vi "Initialize Ref DAQ values.vi"(8 "error in (no error)":errorcluster, 10 "DAQ Input Parameters(FlexRIO)":T2 {"diff_threshZ" format="%#_11g"; "proportioanl_scale Z" format="%#_15g"; "var_x" format="%#_14g"; "var_y" format="%#_14g"; "scale" format="%#_15g"; "diff_thresh" format="%#_11g"; "proportioanl_scale" format="%#_15g"}, 11 "Refnum in":T1) -> (0 "error out":errorcluster, 3 "Refnum out":T1)   [LabVIEW 2020]
uses:
  RIG-SPECIFIC FILES/FPGA Refs/FPGA Ref.ctl
  <vilib>/rvi/interface/nirviReadWriteControl/nirviReadWriteControl.xnode
  <vilib>/rvi/interface/nirviMethod/nirviMethod.xnode
  NiFpgaLv.dll
  <vilib>/Utility/error.llb/Error Cluster From Error Code.vi
  <vilib>/rvi/interface/Simulation/niFpgaSimulationCallBeginRW.vi
  <vilib>/rvi/errors/niLvFpgaAdjustHostInterfaceError.vi
  <vilib>/FPGAPlugInAG/Dynamic/niLvFpga_StartFifo_Dynamic.vi
  <vilib>/rvi/errors/niLvFpgaMergeErrorWithErrorCode.vi
  FPGA DAQ/FPGA Typedefs/scan_typr.ctl
  Movement Correction/Typedefs/Control algorithm.ctl
  Typedefs/Controls/DAQ Input Parameters(FlexRIO).ctl
panel:
  out "scale":fxp<+,16,2>=1.0 format="%#_15g"
  out "New line trigger enabled":bool
  out "Ref count reset enabled":bool
  out "scan_int":fxp<+,16,2>
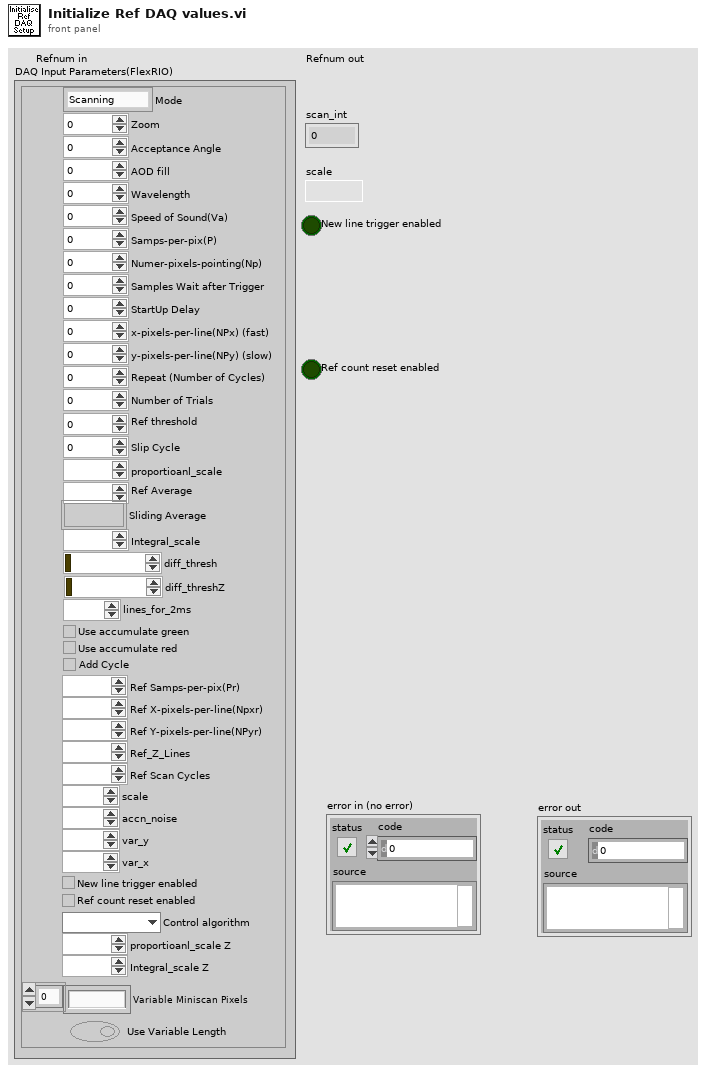
[diagram p1: front panel]
types:
  T1 = typedef "FPGA Ref.ctl" = refnum<k20>
  T2 = typedef "DAQ Input Parameters(FlexRIO).ctl" = cluster{"Mode":T3, "Zoom":i8, "Acceptance Angle":i8, "AOD fill":u16, "Wavelength":i16, "Speed of Sound(Va)":i8, "Samps-per-pix(P)":i16, "Numer-pixels-pointing(Np)":u32, "Samples Wait after Trigger":u16, "StartUp Delay":i32, "x-pixels-per-line(NPx) (fast)":u16, "y-pixels-per-line(NPy) (slow)":u16, "Repeat (Number of Cycles)":u32, "Number of Trials":u16, "Ref threshold":u16, "Slip Cycle":u32, "proportioanl_scale":fxp<+,16,2>, "Ref Average":u16, "Sliding Average":bool, "Integral_scale":fxp<+/-,16,12>, "diff_thresh":fxp<+/-,16,8>, "diff_threshZ":fxp<+/-,16,8>, "lines_for_2ms":i16, "Use accumulate green":bool, "Use accumulate red":bool, "Add Cycle":bool, "Ref Samps-per-pix(Pr)":i16, "Ref X-pixels-per-line(Npxr)":i16, "Ref Y-pixels-per-line(NPyr)":i16, "Ref_Z_Lines":i16, "Ref Scan Cycles":i32, "scale":fxp<+,16,2>, "accn_noise":fxp<+,16,16>, "var_y":fxp<+,16,4>, "var_x":fxp<+,16,4>, "New line trigger enabled":bool, "Ref count reset enabled":bool, "Control algorithm":T4, "proportioanl_scale Z":fxp<+,16,2>, "Integral_scale Z":fxp<+/-,16,12>, "Variable Miniscan Pixels":u16[], "Use Variable Length":bool}
  T3 = typedef "scan_typr.ctl" = enum16{"Scanning", "Pointing", "Pointing & MC", "Scanning & MC"}
  T4 = typedef "Control algorithm.ctl" = enum16{"PID", "Kalman"}
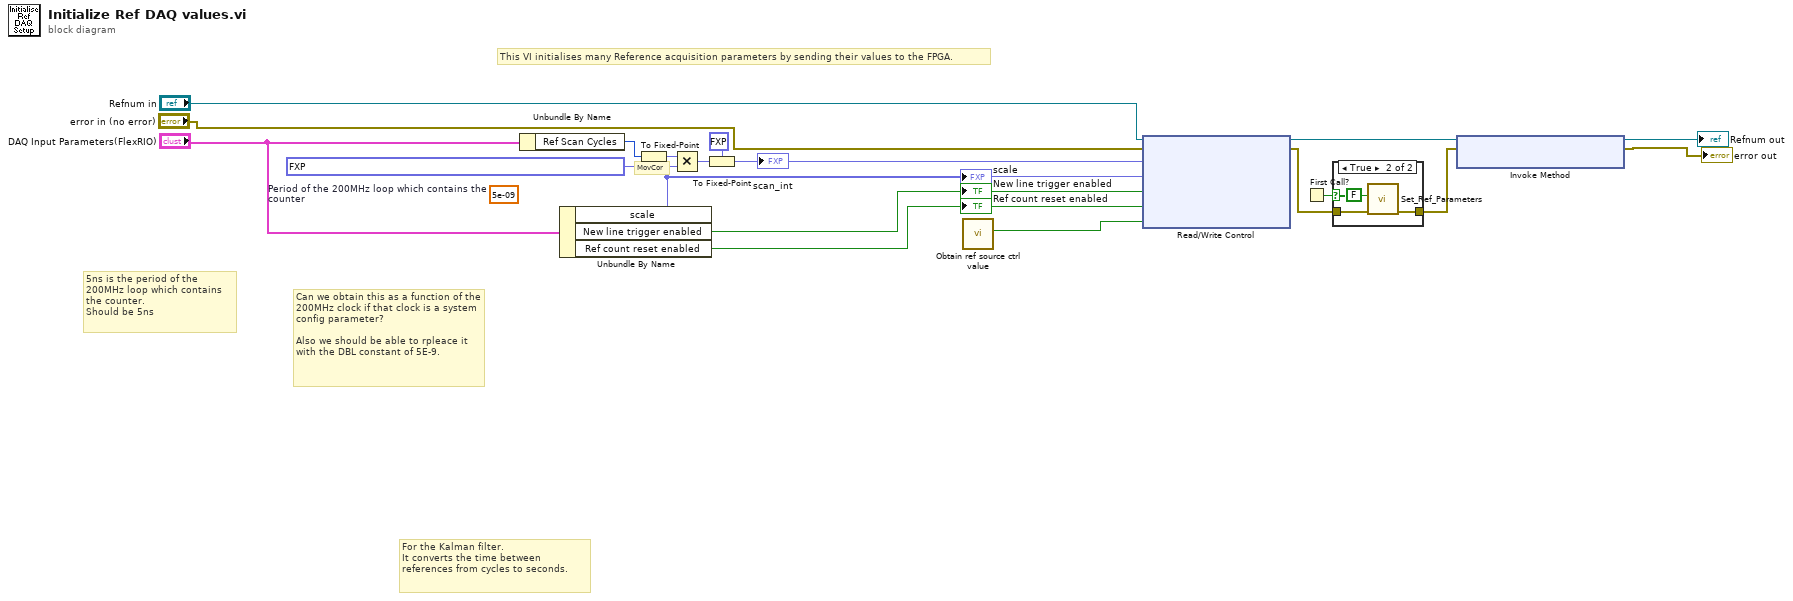
[diagram p0: block diagram]
diagram:
  (unwired) 5e-09  # Period of the 200MHz loop which contains the counter
  # "Can we obtain this as a function of the 200MHz clock if that clock is a system config parameter?\n\nAlso we should be able to rpleace it with the DBL constant of 5E-9."
  # "This VI initialises many Reference acquisition parameters by sending their values to the FPGA."
  # "MovCor"
  # "5ns is the period of the 200MHz loop which contains the counter.\nShould be 5ns"
  # "For the Kalman filter.\nIt converts the time between references from cycles to seconds."
  n1 = Unbundle By Name("DAQ Input Parameters(FlexRIO)") -> ("Ref Scan Cycles"=w12:i32)
  n2 = Unbundle By Name("DAQ Input Parameters(FlexRIO)") -> ("scale"=w14:fxp<+,16,2>, "New line trigger enabled"=w15:bool, "Ref count reset enabled"=w16:bool)
  "Ref count reset enabled" <- w16
  "New line trigger enabled" <- w15
  "scale" <- w14
  n3 = To Fixed-Point(number=w12) -> (fixed-point=w8:fxp<+/-,32,32>)  [unwired: 1 in]
  n4 = Multiply(x=w8, y=fxp<+,64,2> 4.999999999970306e-09 ("fixed-point type")) -> (x*y=w9:fxp<+/-,64,35>)
  n5 = To Fixed-Point(fixed-point type=fxp<+,16,2> 0.0, number=w9) -> (fixed-point=w13:fxp<+,16,2>)
  "scan_int" <- w13
  n6 = call "Obtain ref source ctrl value.vi"() -> ("select_ref_red"=w11:bool)  [unwired: 11 in]
  n7 = xnode ("Read/Write Control")("FPGA VI Reference In"="Refnum in", "error in"="error in (no error)", "scan_int"=w13, "scale"=w14, "New line trigger enabled"=w15, "Ref count reset enabled"=w16, "select_ref_red"=w11) -> ("FPGA VI Reference Out"=w6:T1, "error out"=w5:errorcluster)
  n8 = First Call?() -> (First Call?: T/F=w3:bool)
  n9 = case shown="True" w3 {
    tunnel: w5 -> [w20 w22]
    tunnel: [w20 w21] -> w4
    frame False {
    }
    frame True {
      n10 = call "Set_Ref_Parameters.vi"("error in"=w22, "use_increment_halfrate"=FALSE) -> ("error out"=w21:errorcluster)  [unwired: 7 in, 2 out]
    }
  }
  n11 = xnode ("Invoke Method")("FPGA VI Reference In"=w6, "error in"=w4) -> ("FPGA VI Reference Out"=→"Refnum out":T1, "error out"=→"error out":errorcluster)
